vi "Correlate-time-to-scan-pattern.vi"(0 "Map in":T1, 1 "Read offset":i64, 2 "Camera":string, 3 "Map characteristic":T2, 5 "Pattern time":sgl[](array[numeric]), 7 "Pattern X":sgl[](array[numeric]), 9 "Pattern Y":sgl[](array[numeric]), 11 "error in":errorcluster, 12 "Scan start time [s]":dbl, 13 "Characteristics file ref.":refnum<k34>, 14 "Temperature file ref.":refnum<k34>) -> (4 "Map":T1, 6 "New offset":i64, 15 "error IO":errorcluster)   [LabVIEW 2013, in "CameraVision.lvlib" / "CV-Mapping.lvclass"]
uses:
  CV-Mapping.lvclass
  Mapping-characteristic.ctl
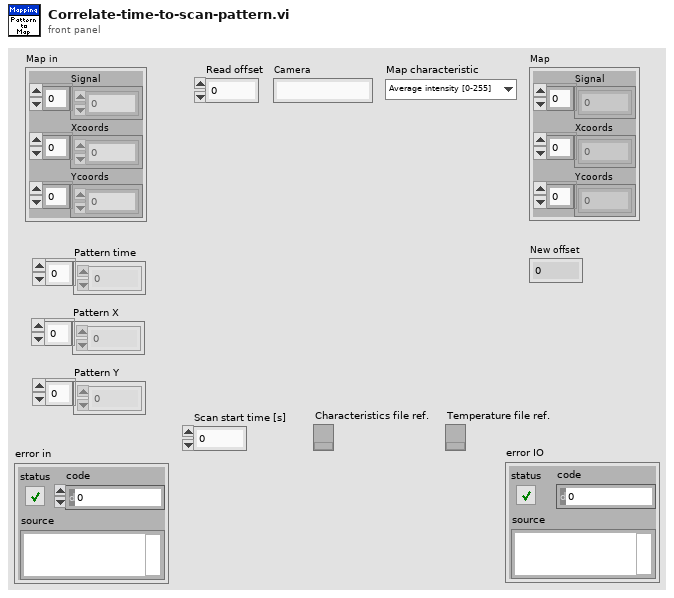
[diagram p1: front panel]
types:
  T1 = cluster{"Signal":sgl[], "Xcoords":sgl[], "Ycoords":sgl[]}
  T2 = typedef "CameraVision.lvlib/CV-Mapping.lvclass/Mapping-characteristic.ctl" = enum16{"Average intensity [0-255]", "Peak intensity [0-255]", "Melt-pool size [mm²]", "Melt-pool aspect ratio []", "Melt-pool fragments []", "Average temperature [°C]", "Max. temperature [°C]", "Min. temperature [°C]", "Std. dev. temperature [°C]"}
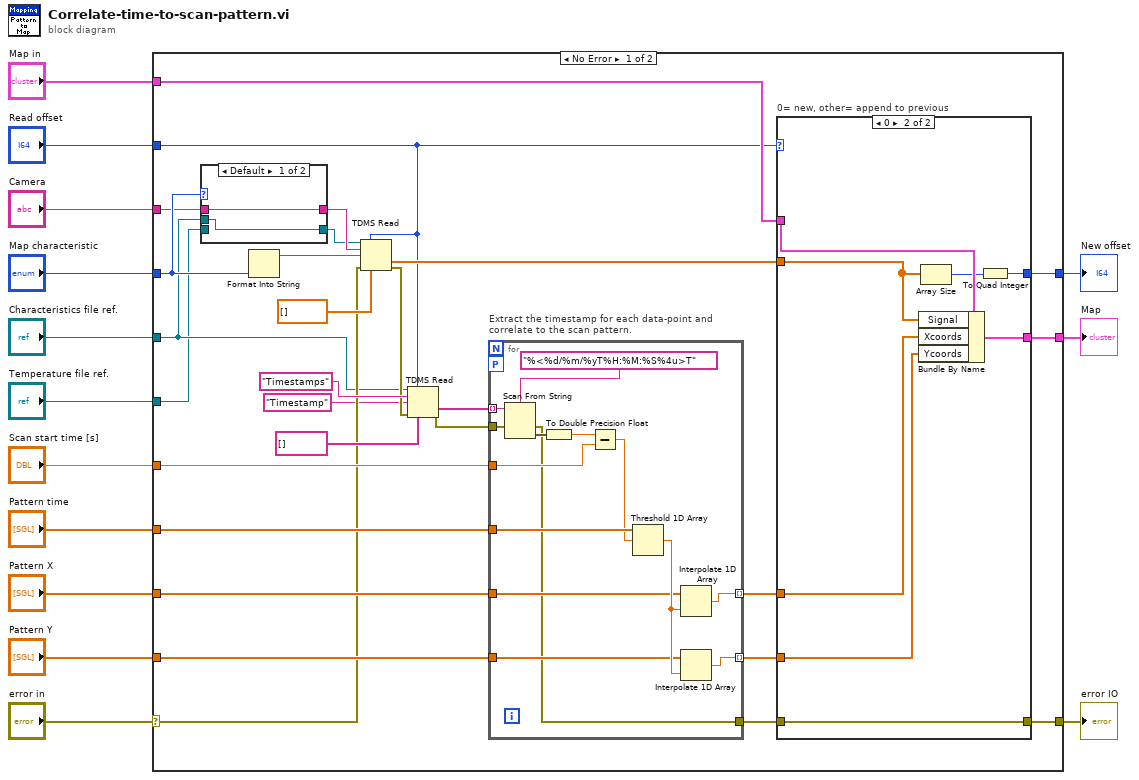
[diagram p0: block diagram]
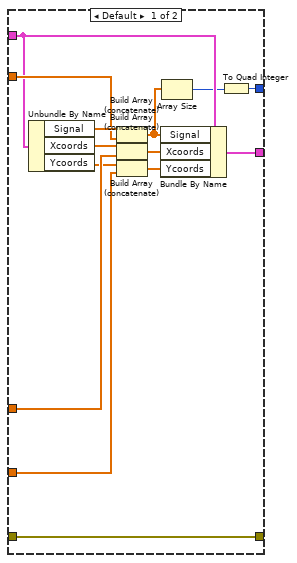
[diagram p2: hidden frame]
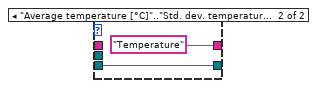
[diagram p3: hidden frame]
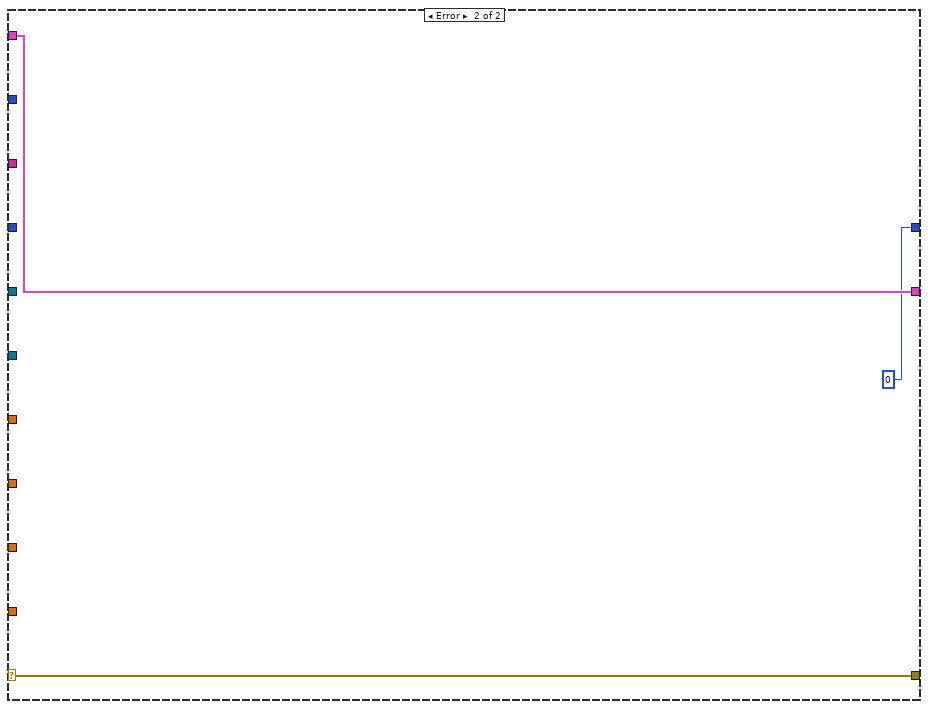
[diagram p4: hidden frame]
diagram:
  n1 = case shown="No Error" "error in" {
    selector: "error in" -> [w32 w85]
    tunnel: "Pattern Y" -> [w42 _]
    tunnel: "Pattern X" -> [w41 _]
    tunnel: "Pattern time" -> [w40 _]
    tunnel: "Read offset" -> [w18 _]
    tunnel: "Scan start time [s]" -> [w38 _]
    tunnel: "Characteristics file ref." -> [w26 _]
    tunnel: "Map characteristic" -> [w33 _]
    tunnel: [w16 w85] -> w8
    tunnel: "Camera" -> [w27 _]
    tunnel: "Temperature file ref." -> [w25 _]
    tunnel: "Map in" -> [w23 w84]
    tunnel: [w17 w84] -> w2
    tunnel: [w15 i64 0] -> w1
    frame No Error {
      n2 = case shown="Default" w33 {
        tunnel: [w66 "Temperature"] -> w35
        tunnel: w27 -> [w66 _]
        tunnel: w26 -> [w65 _]
        tunnel: w25 -> [_ w67]
        tunnel: [w65 w67] -> w24
        frame Default {
        }
        frame "Average temperature [°C]".."Std. dev. temperature [°C]" {
        }
      }
      n3 = Format Into String(w33) -> (resulting string=w34:string)  [unwired: 3 in, 1 out]
      n4 = TDMS Read(0:w24, 1:w18, 5:w35, 7:w34, 11:w32, 12:sgl[] []) -> (10:w19:sgl[], 15:w30:errorcluster)  [unwired: 2 in, 4 out]
      n5 = TDMS Read(0:w26, 1:w18, 5:"Timestamps" ("group name in"), 7:"Timestamp" ("channel name(s) in"), 11:w30, 12:string[] []) -> (10:w28:string[], 15:w31:errorcluster)  [unwired: 2 in, 4 out]
      n6 = for "Extract the timestamp for each data-point and correlate to the scan pattern." {
        tunnel: w28 -> [w70] mode=indexing
        tunnel: w38 -> [w80]
        tunnel: w40 -> [w78]
        tunnel: w41 -> [w77]
        tunnel: w42 -> [w76]
        tunnel: [w74] -> w22 mode=indexing
        tunnel: [w73] -> w21 mode=indexing
        workers-P: _ -> [_]
        tunnel: [w71] -> w20
        tunnel: w31 -> [w72]
        n7 = Scan From String(format string="%<%d/%m/%yT%H:%M:%S%4u>T", input string=w70, error in=w72) -> (error out=w71:errorcluster, output 1=w82:timestamp)  [unwired: 2 in, 2 out]
        n8 = To Double Precision Float(number=w82) -> (double precision float=w81:dbl)
        n9 = Subtract(x=w81, y=w80) -> (x-y=w75:dbl)
        n10 = Threshold 1D Array(2:w75, 3:w78) -> (0:w79:sgl)  [unwired: 1 in]
        n11 = Interpolate 1D Array(1:w79, 2:w77) -> (0:w74:sgl)
        n12 = Interpolate 1D Array(1:w79, 2:w76) -> (0:w73:sgl)
      }
      n13 = case "0= new, other= append to previous" shown="0" w18 {
        tunnel: w23 -> [w49 w64]
        tunnel: w22 -> [w53 w62]
        tunnel: w21 -> [w50 w60]
        tunnel: w20 -> [w47 w61]
        tunnel: w19 -> [w55 w58]
        tunnel: [w48 w63] -> w17
        tunnel: [w47 w61] -> w16
        tunnel: [w45 w59] -> w15
        frame Default {
          n14 = Unbundle By Name(w49) -> ("Signal"=w56:sgl[], "Xcoords"=w54:sgl[], "Ycoords"=w52:sgl[])
          n15 = Build Array (concatenate)(w56, w55) -> (w44:sgl[])
          n16 = Build Array (concatenate)(w54, w53) -> (w51:sgl[])
          n17 = Build Array (concatenate)(w52, w50) -> (w46:sgl[])
          n18 = Bundle By Name(cluster=w49, "Signal"=w44, "Xcoords"=w51, "Ycoords"=w46) -> (w48:T1)
          n19 = Array Size(array=w44) -> (size(s)=w43:i32)
          n20 = To Quad Integer(1:w43) -> (0:w45:i64)
        }
        frame 0 {
          n21 = Bundle By Name(cluster=w64, "Signal"=w58, "Xcoords"=w62, "Ycoords"=w60) -> (w63:T1)
          n22 = Array Size(array=w58) -> (size(s)=w57:i32)
          n23 = To Quad Integer(1:w57) -> (0:w59:i64)
        }
      }
    }
    frame Error {
    }
  }
  "error IO" <- w8
  "Map" <- w2
  "New offset" <- w1
